vi "CHD_TRAJ_BEGIN.vi"   [LabVIEW 2019]
uses:
  CHD_TRAJECTORY_GLOBALS.vi
  <vilib>/Rock Robotics/WPI/ThirdParty/ChoreoLib/ChoreoLib.lvlib
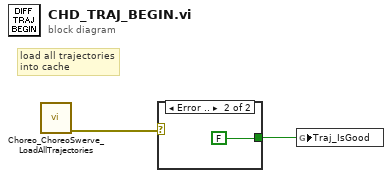
[diagram p0: block diagram]
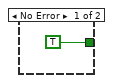
[diagram p2: hidden frame]
diagram:
  # "load all trajectories\ninto cache"
  n1 = call <vilib>:"Choreo_ChoreoSwerve_LoadAllTrajectories.vi"() -> ("error out"=w1:errorcluster)  [unwired: 10 in, 1 out]
  n2 = case shown="Error .." w1 {
    tunnel: [TRUE FALSE] -> w2
    frame No Error {
    }
    frame Error {
    }
  }
  n3 = global write "CHD_TRAJECTORY_GLOBALS.vi" "Traj_IsGood"(w2) -> ()
